vi "Goal Center.vi"(5 "ResolutionY":dbl, 7 "ResolutionX":dbl, 9 "ProjectedY":dbl, 11 "SelectedGoalSubarray":dbl[](array[numeric])) -> (1 "PsuedoJoystickOutPitch":dbl, 3 "PsuedoJoystickOutRotation":dbl)   [LabVIEW 2012]
uses:
  <vilib>/addons/control/pid/pid.llb/PID (DBL).vi
  <vilib>/addons/control/pid/NI_PID_pid.lvlib
panel:
  # "Inputs"
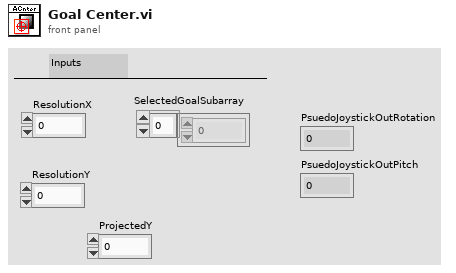
[diagram p1: front panel]
types:
  T1 = cluster{"proportional gain (Kc)":dbl, "integral time (Ti, min)":dbl, "derivative time (Td, min)":dbl}
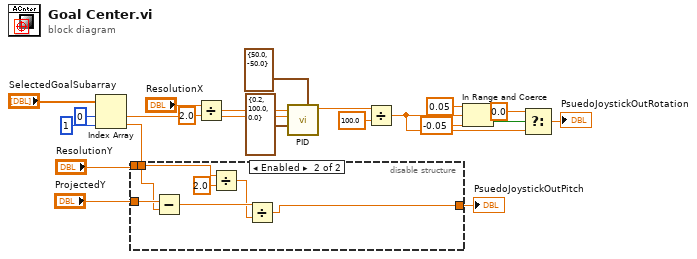
[diagram p0: block diagram]
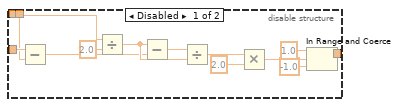
[diagram p2: hidden frame]
diagram:
  n1 = Index Array(array="SelectedGoalSubarray", index #1=0 ("index"), index #2=1 ("index")) -> (element #1=w16:dbl, element #2=w1:dbl)
  n2 = disable-structure shown="Enabled" {
    disable-tunnel: "ResolutionY" -> [w31 w38]
    disable-tunnel: [w27 w35] -> w13
    disable-tunnel: "ProjectedY" -> [w23 w40]
    disable-tunnel: w1 -> [w22 w39]
    frame Disabled {
      n3 = Subtract(x=w23, y=w22) -> (x-y=w24:dbl)
      n4 = Divide(x=w31, y=2.0) -> (x/y=w32:dbl)
      n5 = Subtract(x=w32, y=w24) -> (x-y=w33:dbl)
      n6 = Divide(x=w33, y=w32) -> (x/y=w30:dbl)
      n7 = Multiply(x=w30, y=2.0) -> (x*y=w28:dbl)
      n8 = In Range and Coerce(upper limit=1.0, x=w28, lower limit=-1.0 ("x")) -> (coerced(x)=w27:dbl)  [unwired: 1 out]
    }
    frame Enabled {
      n9 = Subtract(x=w40, y=w39) -> (x-y=w37:dbl)
      n10 = Divide(x=w38, y=2.0) -> (x/y=w36:dbl)
      n11 = Divide(x=w37, y=w36) -> (x/y=w35:dbl)
    }
  }
  "PsuedoJoystickOutPitch" <- w13
  n12 = Divide(x="ResolutionX", y=2.0) -> (x/y=w15:dbl)
  n13 = call-poly <vilib>:"PID.vi"("output range"=cluster{"output high":dbl, "output low":dbl} {"output high"=50.0, "output low"=-50.0}, "PID gains"=T1 {"proportional gain (Kc)"=0.2, "integral time (Ti, min)"=100.0, "derivative time (Td, min)"=0.0}, "process variable"=w16, "setpoint"=w15) -> ("output"=w6:dbl)  [unwired: 6 in, 1 out]
  n14 = Divide(x=w6, y=100.0) -> (x/y=w8:dbl)
  n15 = In Range and Coerce(upper limit=0.05, x=w8, lower limit=-0.05) -> (In Range?=w12:bool)  [unwired: 1 out]
  n16 = Select(t=0.0, s=w12, f=w8) -> (s? t:f=→"PsuedoJoystickOutRotation":dbl)
